vi "ShiftRegister_1.vi"() -> ()   [LabVIEW 2023]
panel:
  in  "stop":bool
  out "Waveform Chart":cluster{dbl, dbl}(graph)
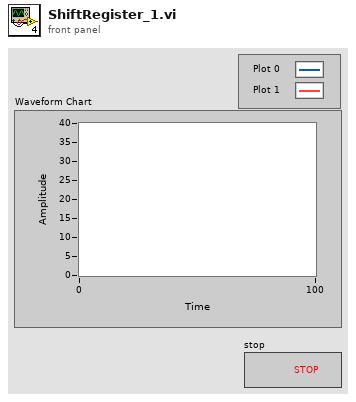
[diagram p1: front panel]
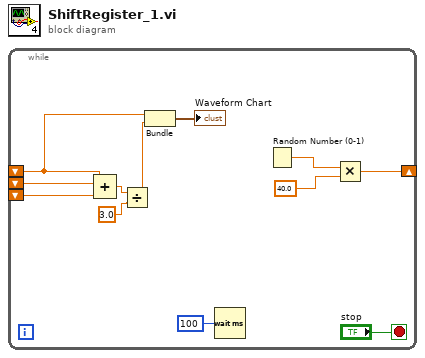
[diagram p0: block diagram]
diagram:
  n1 = while {
    shift-right: [w8] -> _
    shift-left: _ -> [w3]
    shift-left: _ -> [w7]
    shift-left: _ -> [w6]
    stop <- "stop" stop-if-true
    n2 = Compound Arithmetic op=ADD(w3, w7, w6) -> (w5:dbl)
    n3 = Divide(x=w5, y=3.0) -> (x/y=w2:dbl)
    n4 = Bundle(w3, w2) -> (→"Waveform Chart":cluster{dbl, dbl})  [unwired: 1 in]
    n5 = Wait (ms)(milliseconds to wait=u32 100) -> ()  [unwired: 1 out]
    n6 = Random Number (0-1)() -> (number: 0 to 1=w12:dbl)
    n7 = Multiply(x=w12, y=40.0) -> (x*y=w8:dbl)
  }
